vi "Monitor Tool Page.vi"(8 "error in (no error)":errorcluster, 11 "Node Ptr":T1 format="%.0x") -> (0 "error out":errorcluster)   [LabVIEW 2019, in "J1939 Addon System Explorer.lvlib"]
uses:
  J1939 Addon System Explorer.lvlib
  <vilib>/NI VeriStand/Custom Device API/Custom Device Item Ref.ctl
  Addon Shared/Types/Monitor Settings.ctl
  <vilib>/NI VeriStand/Custom Device API/Custom Device API.lvlib
  Addon Shared/J1939 Addon Shared.lvlib
panel:
  in  "Include DA":bool
  in  "Settings":cluster{"Section Name":string}={"Section Name"="J1939 Monitor Tool Settings"}
  in  "J1939 Name":u64 format="%.0x"
  in  "J1939 Network Address":u8 format="%.0x"
  in  "SHDocVw.IWebBrowser2":refnum<k7>(container)
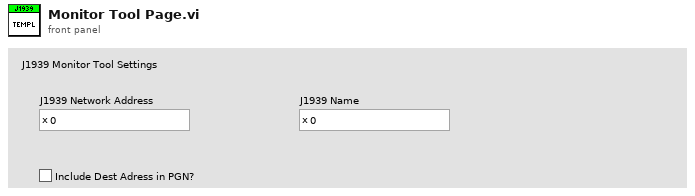
[diagram p1: front panel]
types:
  T1 = typedef "Custom Device API.lvlib/Custom Device Item Ref.ctl" = u64
  T2 = typedef "J1939 Addon Shared.lvlib/Monitor Settings.ctl" = cluster{"Address":u8, "Name":u64, "Include DA":bool}
  T3 = typedef "Custom Device API.lvlib/Custom Device Commands.ctl" = enum16{"Default", "Item renamed", "Shutdown", "Dynamic button pressed"}
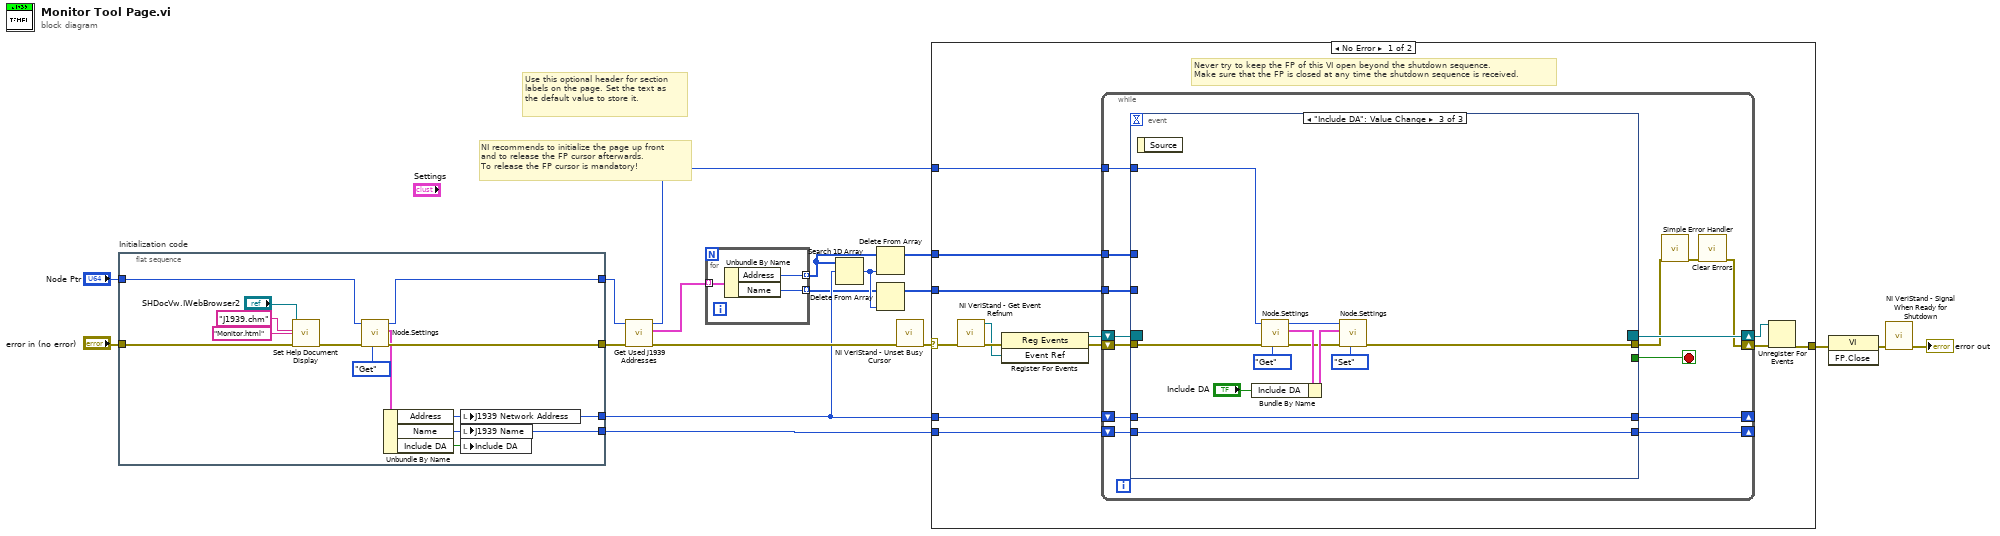
[diagram p0: block diagram]
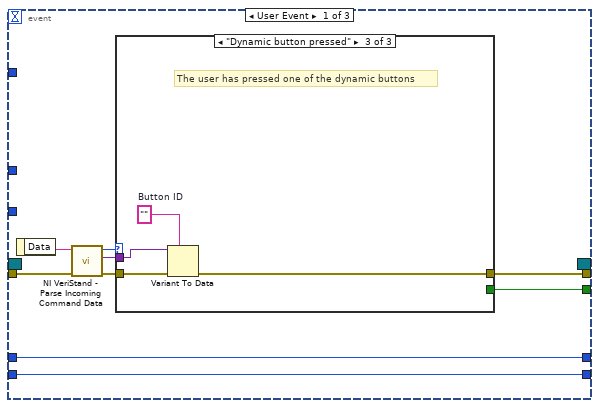
[diagram p2: hidden frame]
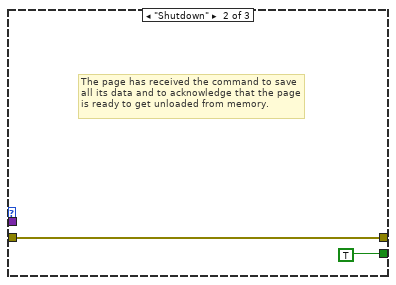
[diagram p4: hidden frame]
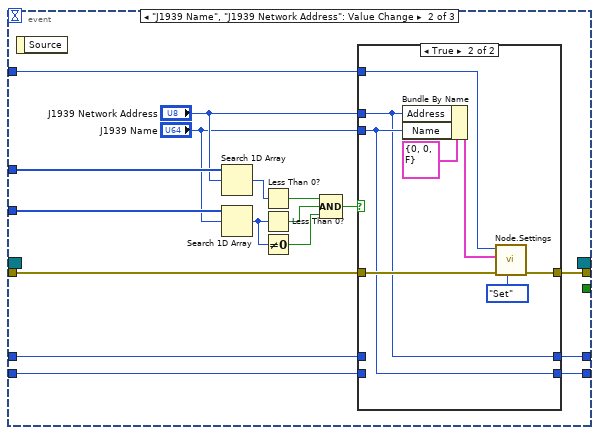
[diagram p5: hidden frame]
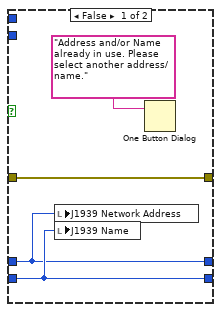
[diagram p6: hidden frame]
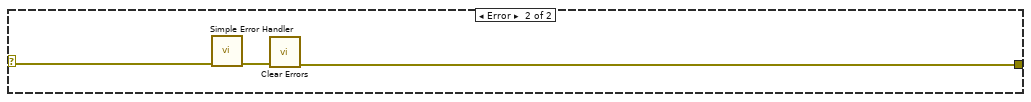
[diagram p7: hidden frame]
diagram:
  # "Use this optional header for section labels on the page. Set the text as the default value to store it."
  # "NI recommends to initialize the page up front\nand to release the FP cursor afterwards.\nTo release the FP cursor is mandatory!"
  n1 = flat-sequence "Initialization code" {
    tunnel: "error in (no error)" -> [w28]
    tunnel: "Node Ptr" -> [w25]
    tunnel: [w23] -> w11
    tunnel: [w21] -> w9
    tunnel: [w27] -> w7
    tunnel: [w26] -> w6
    frame #0 {
      n2 = call "Set Help Document Display.vi"("error in (no error)"=w28, "HTML File"="Monitor.html", "Main CHM File"="J1939.chm", "SHDocVw.IWebBrowser2"="SHDocVw.IWebBrowser2") -> ("error out"=w24:errorcluster)  [unwired: 7 in]
      n3 = call "Node.Settings.vi"("Action"=enum8{"Get", "Set"}."Get", "error in (no error)"=w24, "Item Ref in"=w25) -> ("error out"=w23:errorcluster, "Node.Settings"=w22:T2, "Item Ref out"=w21:T1)  [unwired: 6 in]
      n4 = Unbundle By Name(w22) -> ("Address"=w27:u8, "Name"=w26:u64, "Include DA"=w19:bool)
      n5 = local write "J1939 Network Address"(w27) -> ()
      n6 = local write "J1939 Name"(w26) -> ()
      n7 = local write "Include DA"(w19) -> ()
    }
  }
  n8 = call "Get Used J1939 Addresses.vi"("error in (no error)"=w11, "Node Ptr"=w9) -> ("error out"=w12:errorcluster, "Nodes"=w5:T2[], "Item Ref out"=w10:T1)  [unwired: 7 in]
  n9 = for {
    tunnel: w5 -> [w34] mode=indexing
    tunnel: [w33] -> w4 mode=indexing
    tunnel: [w32] -> w2 mode=indexing
    n10 = Unbundle By Name(w34) -> ("Address"=w33:u8, "Name"=w32:u64)
  }
  n11 = Search 1D Array(1D array=w4, element=w7) -> (index of element=w3:i32)  [unwired: 1 in]
  n12 = Delete From Array(array=w4, index=w3) -> (array with subset deleted=w8:u8[])  [unwired: 1 in, 1 out]
  n13 = Delete From Array(array=w2, index=w3) -> (array with subset deleted=w1:u64[])  [unwired: 1 in, 1 out]
  n14 = call <vilib>:"NI VeriStand - Unset Busy Cursor.vi"("error in (no error)"=w12) -> ("error out"=w14:errorcluster)  [unwired: 10 out]
  n15 = case shown="No Error" w14 {
    selector: w14 -> [w39 w121]
    tunnel: [w44 w119] -> w18
    tunnel: w10 -> [w40 _]
    tunnel: w8 -> [w38 _]
    tunnel: w7 -> [w37 _]
    tunnel: w6 -> [w36 _]
    tunnel: w1 -> [w35 _]
    frame No Error {
      # "Never try to keep the FP of this VI open beyond the shutdown sequence.\nMake sure that the FP is closed at any time the shutdown sequence is received."
      n16 = call <vilib>:"NI VeriStand - Get Event Refnum.vi"("error in (no error)"=w39) -> ("error out"=w47:errorcluster, "Event Ref"=w43:refnum<user-event>)  [unwired: 9 out]
      n17 = register-events(error in=w47, w43) -> (reference out=w41:refnum<event-registration>, error out=w42:errorcluster)  [unwired: 1 in]
      n18 = while {
        tunnel: w40 -> [w57]
        shift-right: [w54] -> w45
        shift-left: w42 -> [w60]
        shift-right: [w61] -> w46
        shift-left: w41 -> [w59]
        tunnel: w38 -> [w53]
        tunnel: w35 -> [w50]
        shift-right: [w48] -> _
        shift-left: w37 -> [w52]
        shift-right: [w49] -> _
        shift-left: w36 -> [w51]
        stop <- w58 stop-if-true
        n19 = event shown="[2] \"Include DA\": Value Change" {
          selector: w59 -> [_ _ _]
          dyn-events: [_ _ _] -> w61
          timeout: _ -> [_ _ _]
          tunnel: w60 -> [w70 w93 w112]
          tunnel: [w66 _ _] -> w58
          tunnel: [w65 w92 w118] -> w56
          tunnel: w57 -> [_ w94 w109]
          tunnel: w53 -> [_ w91 _]
          tunnel: w52 -> [w62 w89 w114]
          tunnel: w51 -> [w63 w88 w115]
          tunnel: w50 -> [_ w87 _]
          tunnel: [w63 w79 w115] -> w49
          tunnel: [w62 w78 w114] -> w48
          event User Event {
            n20 = event-data() -> ("Data"=w69:string)  [unwired: 1 out]
            n21 = call <vilib>:"NI VeriStand - Parse Incoming Command Data.vi"("error in (no error)"=w70, "Incoming data"=w69) -> ("error out"=w68:errorcluster, "Outgoing data"=w64:variant, "Action"=w67:T3)  [unwired: 7 out]
            n22 = case shown="\"Dynamic button pressed\"" w67 {
              tunnel: w68 -> [w71 w72 w77]
              tunnel: [_ TRUE _] -> w66
              tunnel: [w71 w72 w74] -> w65
              tunnel: w64 -> [_ _ w76]
              frame "Default", Default {
              }
              frame "Shutdown" {
                # "The page has received the command to save all its data and to acknowledge that the page is ready to get unloaded from memory."
              }
              frame "Dynamic button pressed" {
                w75 = ""  # Button ID
                # "The user has pressed one of the dynamic buttons"
                n23 = Variant To Data(error in=w77, type=w75, Variant=w76) -> (error out=w74:errorcluster)  [unwired: 1 out]
              }
            }
          }
          event "J1939 Name", "J1939 Network Address": Value Change {
            n24 = event-data() -> ()  [unwired: 2 out]
            n25 = Search 1D Array(1D array=w91, element="J1939 Network Address") -> (index of element=w83:i32)  [unwired: 1 in]
            n26 = Search 1D Array(1D array=w87, element="J1939 Name") -> (index of element=w81:i32)  [unwired: 1 in]
            n27 = Less Than 0?(x=w83) -> (x < 0?=w85:bool)
            n28 = Less Than 0?(x=w81) -> (x < 0?=w84:bool)
            n29 = Not Equal To 0?(x=w81) -> (x != 0?=w80:bool)
            n30 = Compound Arithmetic op=AND(w85, w84, w80) -> (w82:bool)
            n31 = case shown="True" w82 {
              tunnel: w94 -> [_ w106]
              tunnel: w93 -> [w98 w105]
              tunnel: [w98 w104] -> w92
              tunnel: "J1939 Network Address" -> [_ w101]
              tunnel: "J1939 Name" -> [_ w102]
              tunnel: w89 -> [w95 _]
              tunnel: w88 -> [w96 _]
              tunnel: [w96 w102] -> w79
              tunnel: [w95 w101] -> w78
              frame False {
                n32 = local write "J1939 Network Address"(w95) -> ()
                n33 = local write "J1939 Name"(w96) -> ()
                n34 = One Button Dialog(message="Address and/or Name already in use. Please select another address/name.") -> ()  [unwired: 1 in, 1 out]
              }
              frame True {
                n35 = Bundle By Name(cluster=T2 {"Address"=0, "Name"=0, "Include DA"=FALSE} ("J1939 XNET Settings"), "Address"=w101, "Name"=w102) -> (w100:T2)
                n36 = call "Node.Settings.vi"("Action"=enum8{"Get", "Set"}."Set", "error in (no error)"=w105, "Node.Settings"=w100, "Item Ref in"=w106) -> ("error out"=w104:errorcluster)  [unwired: 5 in, 2 out]
              }
            }
          }
          event "Include DA": Value Change {
            n37 = event-data() -> ()  [unwired: 2 out]
            n38 = call "Node.Settings.vi"("Action"=enum8{"Get", "Set"}."Get", "error in (no error)"=w112, "Item Ref in"=w109) -> ("error out"=w110:errorcluster, "Node.Settings"=w111:T2, "Item Ref out"=w108:T1)  [unwired: 6 in]
            n39 = Bundle By Name(cluster=w111, "Include DA"="Include DA") -> (w117:T2)
            n40 = call "Node.Settings.vi"("Action"=enum8{"Get", "Set"}."Set", "error in (no error)"=w110, "Node.Settings"=w117, "Item Ref in"=w108) -> ("error out"=w118:errorcluster)  [unwired: 5 in, 2 out]
          }
        }
        n41 = call <vilib>:"Simple Error Handler.vi"("error in (no error)"=w56) -> ("error out"=w55:errorcluster)  [unwired: 1 in, 7 out]
        n42 = call <vilib>:"Clear Errors.vi"("error in (no error)"=w55) -> ("error out"=w54:errorcluster)  [unwired: 1 in, 5 out]
      }
      n43 = Unregister For Events(event registration refnum=w46, error in=w45) -> (error out=w44:errorcluster)
    }
    frame Error {
      n44 = call <vilib>:"Simple Error Handler.vi"("error in (no error)"=w121) -> ("error out"=w120:errorcluster)  [unwired: 1 in, 7 out]
      n45 = call <vilib>:"Clear Errors.vi"("error in (no error)"=w120) -> ("error out"=w119:errorcluster)  [unwired: 1 in, 5 out]
    }
  }
  n46 = invoke class="VI" method="FP.Close"(error in=w18) -> (error out=w17:errorcluster)  [unwired: 2 in, 2 out]
  n47 = call <vilib>:"NI VeriStand - Signal When Ready for Shutdown.vi"("error in (no error)"=w17) -> ("error out"=→"error out":errorcluster)  [unwired: 10 out]
